vi "read_estimators.vi"(8 "error in (no error)":errorcluster, 11 "StackingClassifier in":refnum<class "StackingClassifier.lvclass">) -> (0 "error out":errorcluster, 2 "params.estimators":string[](array[string]), 3 "StackingClassifier out":refnum<class "StackingClassifier.lvclass">)   [LabVIEW 2020, in "StackingClassifier.lvclass"]
uses:
  StackingClassifier.lvclass
  StackingClassifier.lvclass/StackingClassifier.ctl
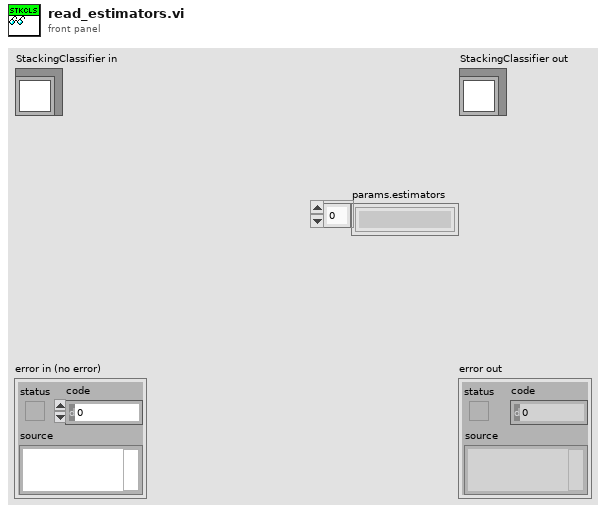
[diagram p1: front panel]
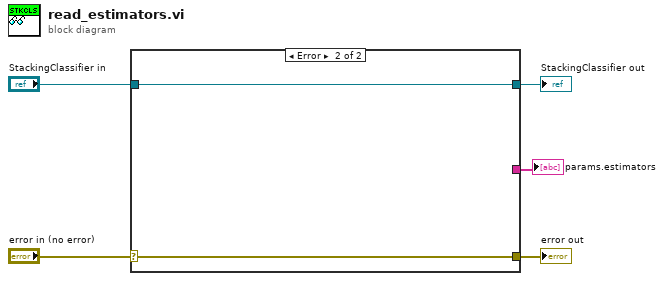
[diagram p0: block diagram]
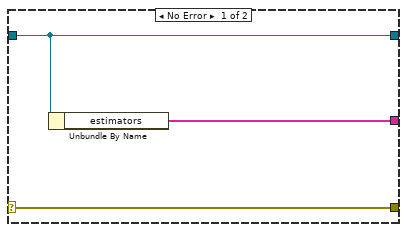
[diagram p2: hidden frame]
diagram:
  n1 = case shown="Error" "error in (no error)" {
    selector: "error in (no error)" -> [w8 w9]
    tunnel: [w8 w9] -> w4
    tunnel: [w7 w10] -> w2
    tunnel: "StackingClassifier in" -> [w7 w10]
    tunnel: [w6 _] -> w1
    frame No Error {
      n2 = Unbundle By Name(w7) -> ("estimators"=w6:string[])
    }
    frame Error {
    }
  }
  "error out" <- w4
  "StackingClassifier out" <- w2
  "params.estimators" <- w1
